vi "Handle Command.vi"(8 "error in (no error)":errorcluster, 9 "Value":bool, 11 "Valve in":refnum<class "DiscreteRangeControl.lvclass">) -> (0 "error out":errorcluster, 3 "Valve out":refnum<class "DiscreteRangeControl.lvclass">)   [LabVIEW 2020, in "VolatusControl.lvlib" / "DiscreteRangeControl.lvclass"]
uses:
  DiscreteRangeControl.lvclass
  DiscreteRangeControl.lvclass/DiscreteRangeControl.ctl
  State.ctl
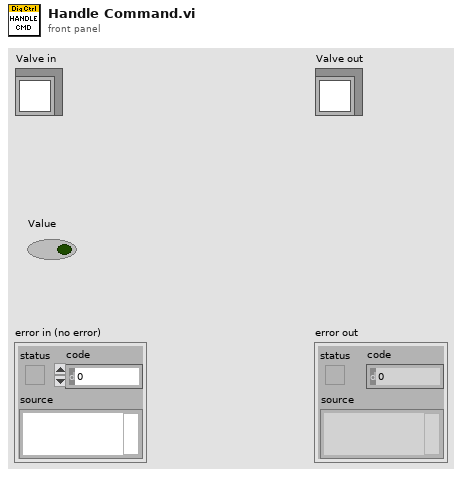
[diagram p1: front panel]
types:
  T1 = typedef "VolatusControl.lvlib/DiscreteRangeControl.lvclass/State.ctl" = enum16{"Idle", "Start", "Run", "Stop"}
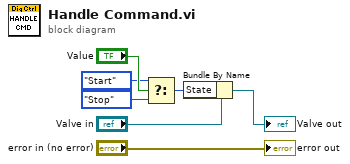
[diagram p0: block diagram]
diagram:
  n1 = Select(t=State."Start" ("State"), s="Value", f=State."Stop" ("State")) -> (s? t:f=w1:T1)
  n2 = Bundle By Name(cluster="Valve in", "State"=w1) -> (→"Valve out":refnum<class "DiscreteRangeControl.lvclass">)
  "error out" <- "error in (no error)"
